vi "init control__polymorphic.vi"   [LabVIEW 2010, in "Control.lvclass"]
uses:
  Control.lvclass
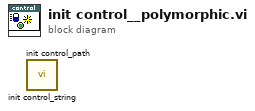
[diagram p0: block diagram]
diagram:
  n1 = call "init control_string.vi"() -> ()  [unwired: 11 in, 1 out]
  n2 = call "init control_path.vi"() -> ()  [unwired: 11 in, 1 out]
